vi "Stepper control.vi"(5 "Error":dbl, 7 "Timer":dbl, 8 "Pos 0":dbl, 11 "Pos +":dbl) -> (0 "Pos":dbl, 1 "Dir":bool, 2 "Frequency":dbl, 3 "Duty Cycle":dbl)   [LabVIEW 2017]
panel:
  in  "Speed":dbl=1000.0
  in  "Hz Limit":dbl
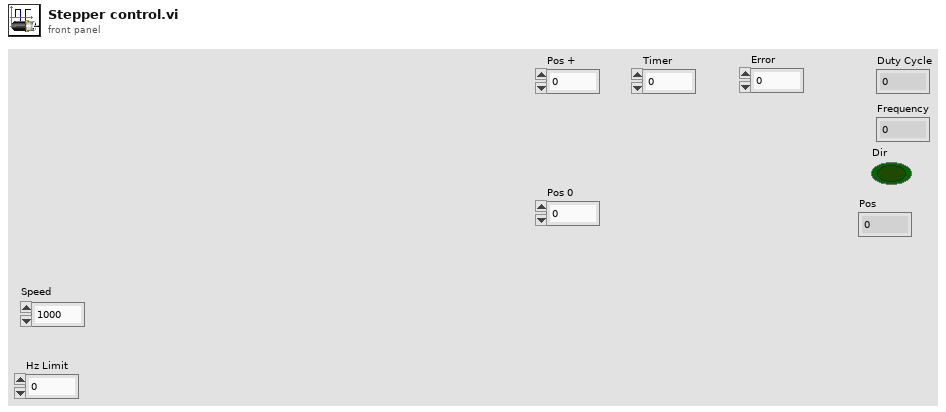
[diagram p1: front panel]
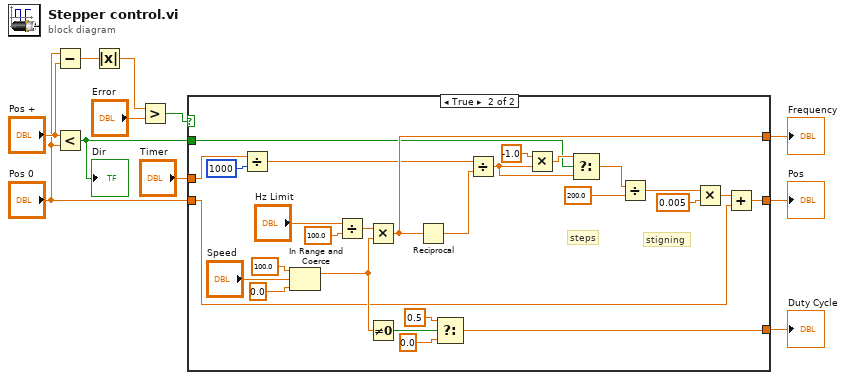
[diagram p0: block diagram]
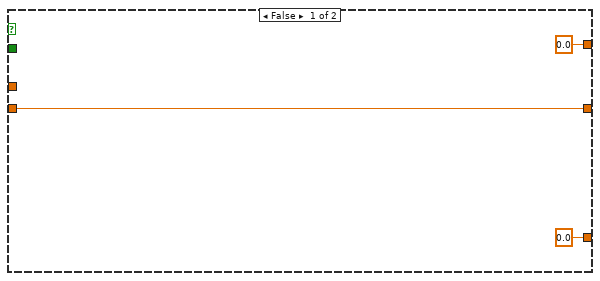
[diagram p2: hidden frame]
diagram:
  n1 = Subtract(x="Pos 0", y="Pos +") -> (x-y=w11:dbl)
  n2 = Less?(x="Pos +", y="Pos 0") -> (x < y?=w5:bool)
  "Dir" <- w5
  n3 = Absolute Value(x=w11) -> (abs(x)=w9:dbl)
  n4 = Greater?(x=w9, y="Error") -> (0:w10:bool)
  n5 = case shown="True" w10 {
    tunnel: [0.0 ("f") w41] -> w6
    tunnel: [0.0 w30] -> w7
    tunnel: "Timer" -> [_ w29]
    tunnel: "Pos 0" -> [w14 w25]
    tunnel: w5 -> [_ w21]
    tunnel: [w14 w20] -> w8
    frame False {
    }
    frame True {
      # "steps"
      # "stigning"
      n6 = Divide(x=w29, y=u32 1000) -> (x/y=w27:dbl)
      n7 = In Range and Coerce(upper limit=100.0, x="Speed", lower limit=0.0) -> (coerced(x)=w31:dbl)  [unwired: 1 out]
      n8 = Divide(x="Hz Limit", y=100.0) -> (x/y=w32:dbl)
      n9 = Multiply(x=w32, y=w31) -> (x*y=w30:dbl)
      n10 = Not Equal To 0?(x=w31) -> (x != 0?=w40:bool)
      n11 = Reciprocal(x=w30) -> (1/x=w26:dbl)
      n12 = Select(t=0.5, s=w40, f=0.0) -> (s? t:f=w41:dbl)
      n13 = Divide(x=w27, y=w26) -> (x/y=w23:dbl)
      n14 = Multiply(x=-1.0, y=w23) -> (x*y=w24:dbl)
      n15 = Select(t=w24, s=w21, f=w23) -> (s? t:f=w18:dbl)
      n16 = Divide(x=w18, y=200.0) -> (x/y=w17:dbl)
      n17 = Multiply(x=w17, y=0.005) -> (x*y=w16:dbl)
      n18 = Add(x=w16, y=w25) -> (x+y=w20:dbl)
    }
  }
  "Duty Cycle" <- w6
  "Frequency" <- w7
  "Pos" <- w8
